vi "__SBR_Ana2.vi"(9 "SBRAクラスタ":T1={"データ配列"=array801x21[16821 elements], "Points"=801, "Th"=297.0, "Tc"=77.0, "LO(GHz)"=920.0, "Offset(mm)"=23.113, "Pos(mm)"=0.0, "P/V         V/P"=FALSE, "AUTOSAVE"=TRUE, "file_name"="", "パス"=path "", "header+(filename)"="A_"}) -> (0 "XYグラフ 6":cluster{"データ配列":dbl[], "データ配列":dbl[]}[](graph), 2 "XYグラフ 9":cluster{"データ配列":dbl[], "データ配列":dbl[]}[](graph), 3 "XYグラフ 5":cluster{"データ配列":dbl[], "データ配列":dbl[]}[](graph))   [LabVIEW 2017]
uses:
  <vilib>/Utility/file.llb/Read From Spreadsheet File (DBL).vi
  <vilib>/express/express arith-compare/Formula/XNode/ExpressFormulaBlockNode.xnode
panel:
  out "XYグラフ 8":cluster{"データ配列":dbl[], "データ配列":dbl[]}[](graph)
  in  "タブ制御器":T2(tab)
  out "XYグラフ":cluster{dbl[], dbl[]}[](graph)
  out "XYグラフ 4":cluster{"データ配列":dbl[], "データ配列":dbl[]}[](graph)
  out "XYグラフ 7":cluster{"データ配列":dbl[], "データ配列":dbl[]}[](graph)
  # "Port"
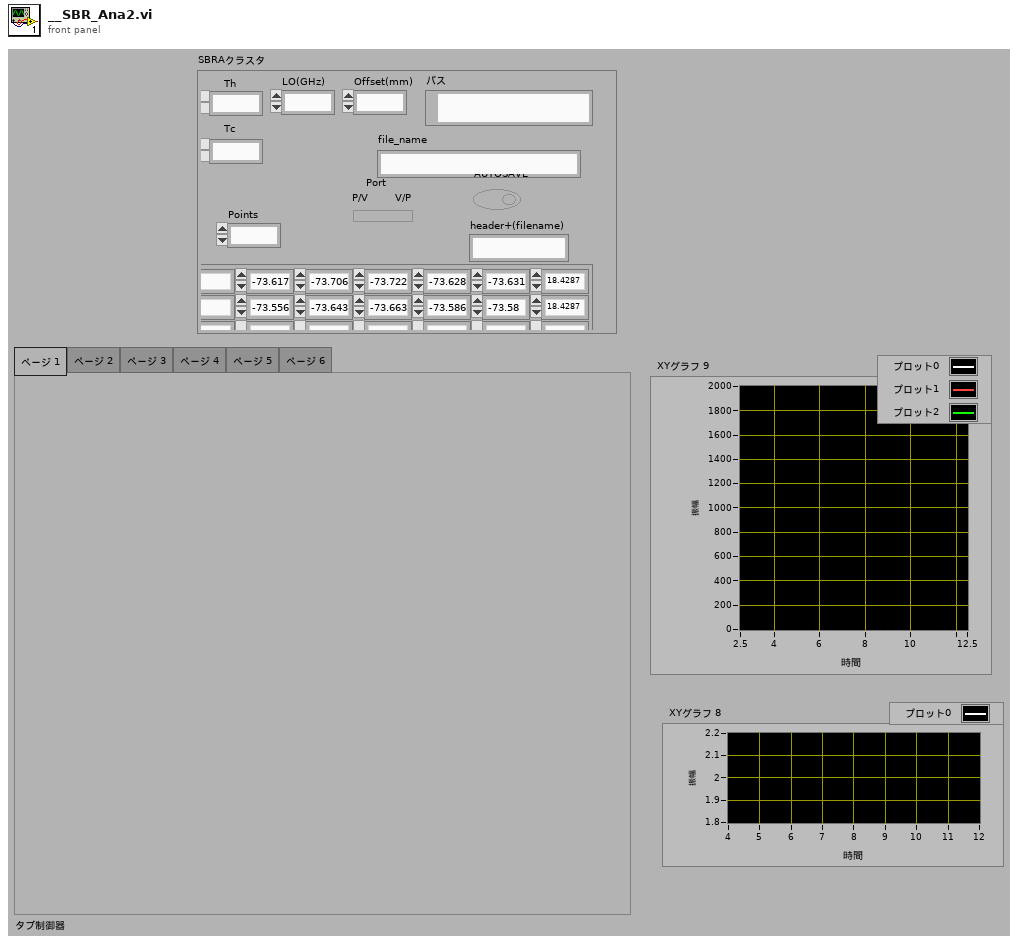
[diagram p1: front panel]
types:
  T1 = cluster{"データ配列":dbl[][], "Points":i32, "Th":dbl, "Tc":dbl, "LO(GHz)":dbl, "Offset(mm)":dbl, "Pos(mm)":dbl, "P/V         V/P":bool, "AUTOSAVE":bool, "file_name":string, "パス":path, "header+(filename)":string}
  T2 = enum32{"ページ 1", "ページ 2", "ページ 3", "ページ 4", "ページ 5", "ページ 6"}
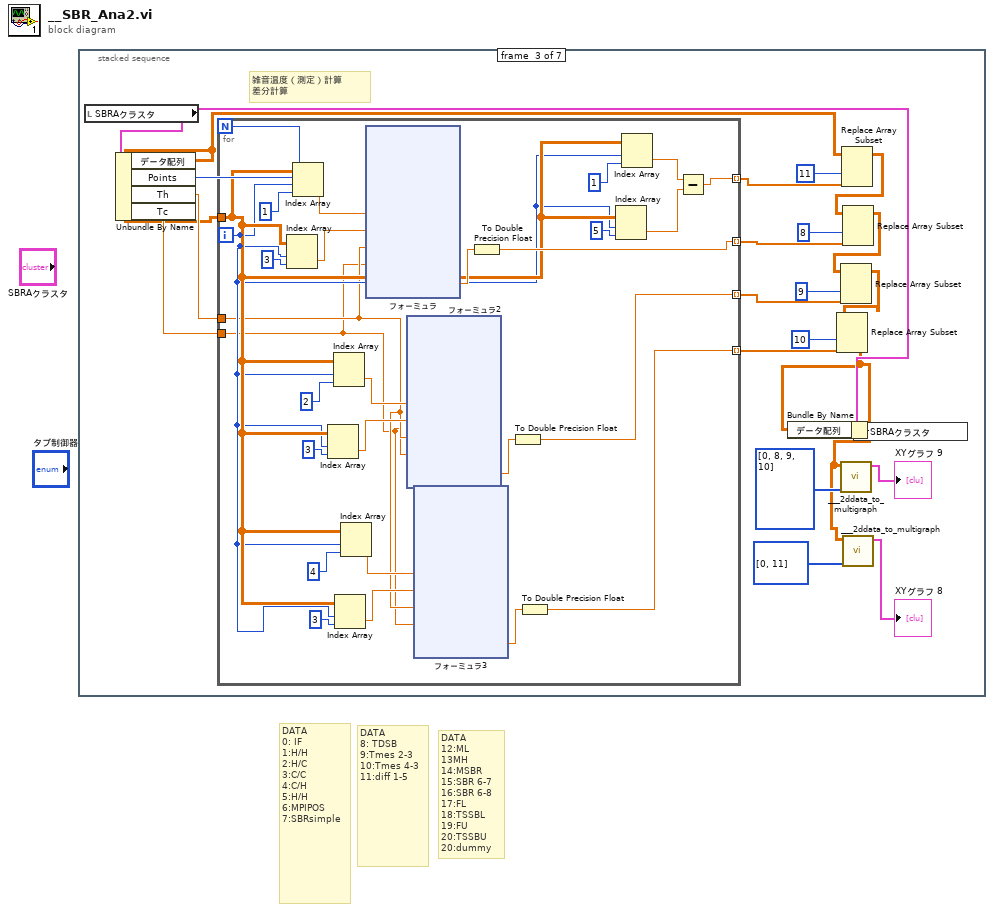
[diagram p0: block diagram]
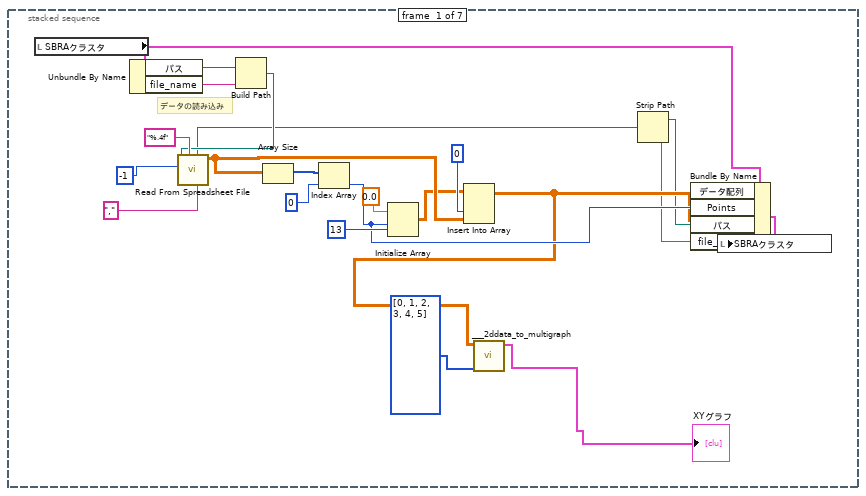
[diagram p2: hidden frame]
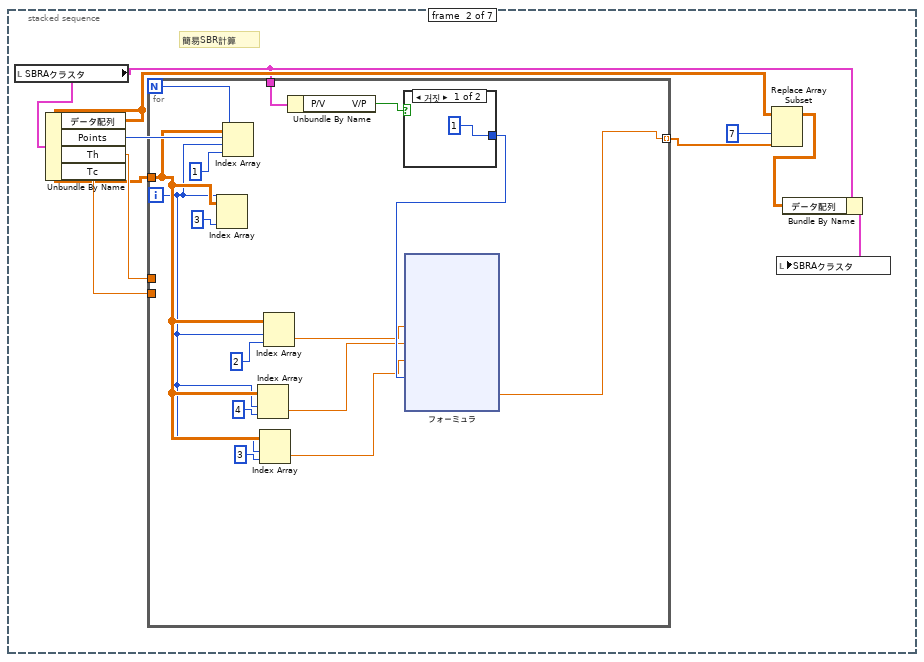
[diagram p3: hidden frame]
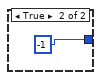
[diagram p4: hidden frame]
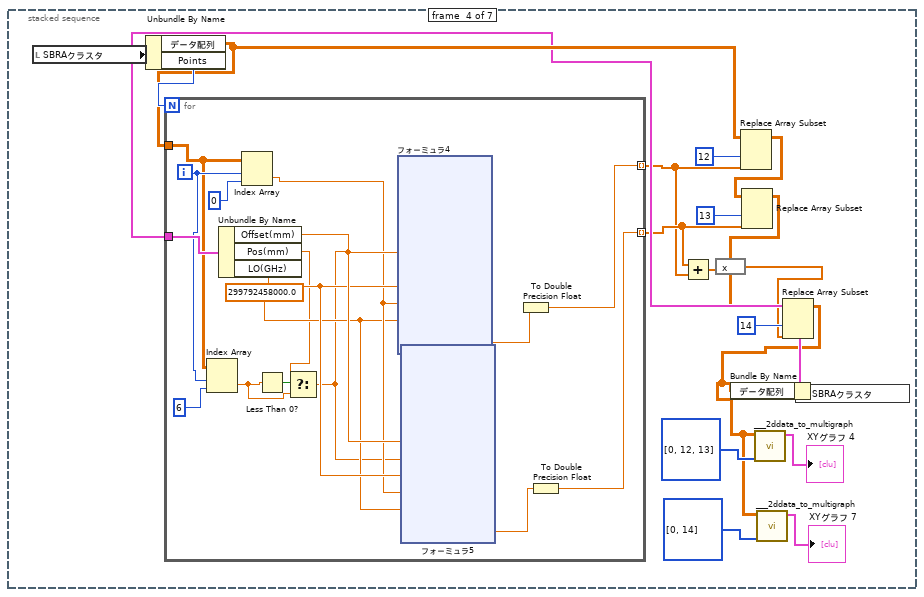
[diagram p5: hidden frame]
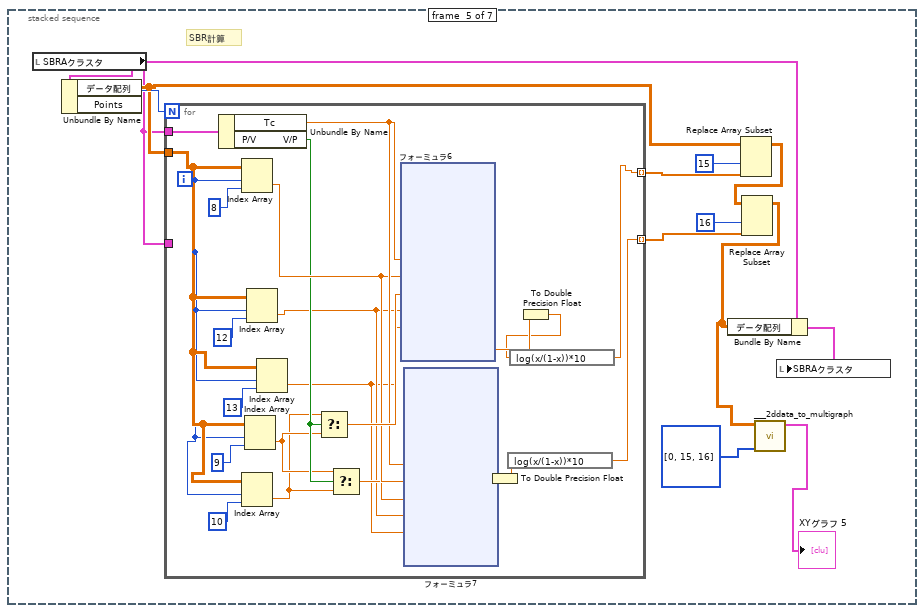
[diagram p6: hidden frame]
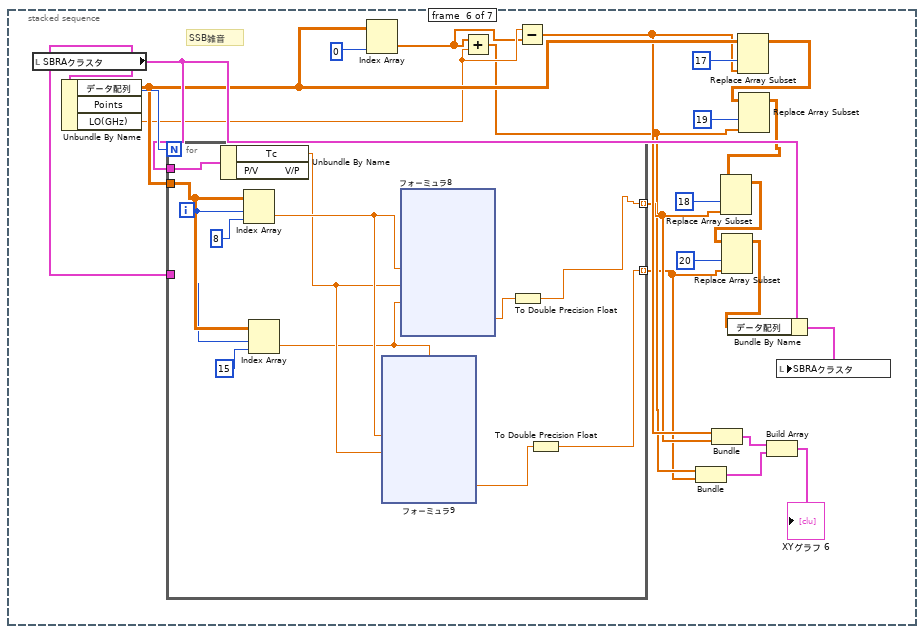
[diagram p7: hidden frame]
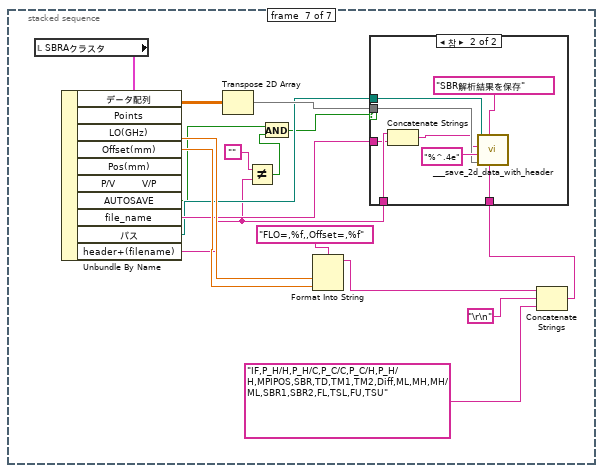
[diagram p8: hidden frame]
diagram:
  # "DATA\n12:ML\n13MH\n14:MSBR\n15:SBR 6-7\n16:SBR 6-8\n17:FL\n18:TSSBL\n19:FU\n20:TSSBU\n20:dummy"
  # "DATA\n8: TDSB\n9:Tmes 2-3\n10:Tmes 4-3\n11:diff 1-5"
  # "DATA\n0: IF\n1:H/H\n2:H/C\n3:C/C\n4:C/H\n5:H/H\n6:MPIPOS\n7:SBRsimple"
  n1 = stacked-sequence {
    frame #0 {
      # "データの読み込み"
      n2 = local read "SBRAクラスタ"() -> (w7:T1)
      n3 = Unbundle By Name(w7) -> ("パス"=w6:path, "file_name"=w5:string)
      n4 = Build Path(base path=w6, name or relative path=w5) -> (appended path=w4:path)
      n5 = call-poly <vilib>:"Read From Spreadsheet File.vi"("delimiter (\\t)"=",", "format (%.3f)"="%.4f", "number of rows (all:-1)"=-1, "file path (dialog if empty)"=w4) -> ("all rows"=w9:dbl[][], "new file path (Not A Path if cancelled)"=w1:path)  [unwired: 3 in, 3 out]
      n6 = Array Size(array=w9) -> (size(s)=w20:i32[])
      n7 = Index Array(array=w20, index=0) -> (element=w14:i32)
      n8 = Initialize Array(0.0, w14, 13) -> (w8:dbl[][])
      n9 = Insert Into Array(array=w8, index (col)=0, new element=w9) -> (w12:dbl[][])  [unwired: 1 in]
      n10 = call "___2ddata_to_multigraph.vi"("列"=i32[] [0, 1, 2, 3, 4, 5], "データ配列"=w12) -> ("XYグラフ"=→"XYグラフ":cluster{"データ配列":dbl[], "データ配列":dbl[]}[])  [unwired: 5 in]
      n11 = Strip Path(path=w1) -> (stripped path=w3:path, name=w2:string)
      n12 = Bundle By Name(cluster=w7, "データ配列"=w12, "Points"=w14, "パス"=w3, "file_name"=w2) -> (w15:T1)
      n13 = local write "SBRAクラスタ"(w15) -> ()
    }
    frame #1 {
      # "簡易SBR計算"
      n14 = local read "SBRAクラスタ"() -> (w24:T1)
      n15 = Unbundle By Name(w24) -> ("データ配列"=w28:dbl[][], "Points"=w31:i32, "Th"=w30:dbl, "Tc"=w29:dbl)
      n16 = for {
        N: w31 -> [_]
        tunnel: w28 -> [w40]
        tunnel: w30 -> [_]
        tunnel: w29 -> [_]
        tunnel: [w32] -> w25 mode=indexing
        tunnel: w24 -> [w38]
        i -> [w39]
        n17 = Index Array(array=w40, index (row)=w39, index (col)=3) -> ()  [unwired: 1 out]
        n18 = Index Array(array=w40, index (row)=w39, index (col)=1) -> ()  [unwired: 1 out]
        n19 = Index Array(array=w40, index (row)=w39, index (col)=4) -> (element=w34:dbl)
        n20 = Index Array(array=w40, index (row)=w39, index (col)=3) -> (element=w33:dbl)
        n21 = Index Array(array=w40, index (row)=w39, index (col)=2) -> (element=w35:dbl)
        n22 = Unbundle By Name(w38) -> ("P/V         V/P"=w37:bool)
        n23 = case shown="거짓" w37 {
          tunnel: [1 -1] -> w36
          frame False {
          }
          frame True {
          }
        }
        n24 = xnode "フォーミュラ"("PHC"=w35, "PCH"=w34, "PCC"=w33, "sig"=w36) -> ("結果"=w32:dbl)  [unwired: 1 in, 1 out]
      }
      n25 = Replace Array Subset(array=w28, new element=w25, index (col)=7) -> (w23:dbl[][])  [unwired: 1 in]
      n26 = Bundle By Name(cluster=w24, "データ配列"=w23) -> (w27:T1)
      n27 = local write "SBRAクラスタ"(w27) -> ()
    }
    frame #2 {
      # "雑音温度（測定）計算\n差分計算"
      n28 = local read "SBRAクラスタ"() -> (w79:T1)
      n29 = Unbundle By Name(w79) -> ("データ配列"=w80:dbl[][], "Points"=w83:i32, "Th"=w82:dbl, "Tc"=w81:dbl)
      n30 = for {
        N: w83 -> [_]
        tunnel: [w109] -> w73 mode=indexing
        tunnel: w80 -> [w92]
        tunnel: w82 -> [w85]
        tunnel: w81 -> [w84]
        tunnel: [w89] -> w76 mode=indexing
        tunnel: [w87] -> w68 mode=indexing
        tunnel: [w86] -> w67 mode=indexing
        i -> [w88]
        n31 = Index Array(array=w92, index (row)=w88, index (col)=3) -> (element=w106:dbl)
        n32 = Index Array(array=w92, index (row)=w88, index (col)=1) -> (element=w105:dbl)
        n33 = Index Array(array=w92, index (row)=w88, index (col)=3) -> (element=w101:dbl)
        n34 = Index Array(array=w92, index (row)=w88, index (col)=2) -> (element=w100:dbl)
        n35 = Index Array(array=w92, index (row)=w88, index (col)=3) -> (element=w96:dbl)
        n36 = Index Array(array=w92, index (row)=w88, index (col)=4) -> (element=w95:dbl)
        n37 = xnode "フォーミュラ"("ph"=w105, "pc"=w106, "th"=w85, "tc"=w84) -> ("結果"=w110:dbl)  [unwired: 1 in, 1 out]
        n38 = xnode "フォーミュラ2"("ph"=w100, "pc"=w101, "th"=w85, "tc"=w84) -> ("結果"=w104:dbl)  [unwired: 1 in, 1 out]
        n39 = xnode "フォーミュラ3"("ph"=w95, "pc"=w96, "th"=w85, "tc"=w84) -> ("結果"=w99:dbl)  [unwired: 1 in, 1 out]
        n40 = To Double Precision Float(number=w110) -> (double precision float=w109:dbl)
        n41 = To Double Precision Float(number=w104) -> (double precision float=w87:dbl)
        n42 = To Double Precision Float(number=w99) -> (double precision float=w86:dbl)
        n43 = Index Array(array=w92, index (row)=w88, index (col)=5) -> (element=w90:dbl)
        n44 = Index Array(array=w92, index (row)=w88, index (col)=1) -> (element=w91:dbl)
        n45 = Subtract(x=w91, y=w90) -> (x-y=w89:dbl)
      }
      n46 = Replace Array Subset(array=w80, new element=w76, index (col)=11) -> (w74:dbl[][])  [unwired: 1 in]
      n47 = Replace Array Subset(array=w74, new element=w73, index (col)=8) -> (w71:dbl[][])  [unwired: 1 in]
      n48 = Replace Array Subset(array=w71, new element=w68, index (col)=9) -> (w69:dbl[][])  [unwired: 1 in]
      n49 = Replace Array Subset(array=w69, new element=w67, index (col)=10) -> (w63:dbl[][])  [unwired: 1 in]
      n50 = Bundle By Name(cluster=w79, "データ配列"=w63) -> (w78:T1)
      n51 = call "___2ddata_to_multigraph.vi"("列"=i32[] [0, 8, 9, 10], "データ配列"=w63) -> ("XYグラフ"=→"XYグラフ 9":cluster{"データ配列":dbl[], "データ配列":dbl[]}[])  [unwired: 5 in]
      n52 = call "___2ddata_to_multigraph.vi"("列"=i32[] [0, 11], "データ配列"=w63) -> ("XYグラフ"=→"XYグラフ 8":cluster{"データ配列":dbl[], "データ配列":dbl[]}[])  [unwired: 5 in]
      n53 = local write "SBRAクラスタ"(w78) -> ()
    }
    frame #3 {
      n54 = local read "SBRAクラスタ"() -> (w165:T1)
      n55 = Unbundle By Name(w165) -> ("データ配列"=w166:dbl[][], "Points"=w170:i32)
      n56 = for {
        N: w170 -> [_]
        tunnel: w166 -> [w175]
        tunnel: w165 -> [w186]
        tunnel: [w179] -> w160 mode=indexing
        tunnel: [w178] -> w161 mode=indexing
        i -> [w176]
        w182 = 299792458000.0
        n57 = Index Array(array=w175, index (row)=w176, index (col)=6) -> (element=w172:dbl)
        n58 = Unbundle By Name(w186) -> ("Offset(mm)"=w185:dbl, "Pos(mm)"=w173:dbl, "LO(GHz)"=w184:dbl)
        n59 = Index Array(array=w175, index (row)=w176, index (col)=0) -> (element=w183:dbl)
        n60 = Less Than 0?(x=w172) -> (x < 0?=w174:bool)
        n61 = Select(t=w173, s=w174, f=w172) -> (s? t:f=w171:dbl)
        n62 = xnode "フォーミュラ4"("OS"=w185, "POS"=w171, "LO"=w184, "IF"=w183, "VC"=w182) -> ("結果"=w181:dbl)  [unwired: 1 in, 1 out]
        n63 = xnode "フォーミュラ5"("OS"=w185, "POS"=w171, "LO"=w184, "IF"=w183, "VC"=w182) -> ("結果"=w180:dbl)  [unwired: 1 in, 1 out]
        n64 = To Double Precision Float(number=w181) -> (double precision float=w179:dbl)
        n65 = To Double Precision Float(number=w180) -> (double precision float=w178:dbl)
      }
      n66 = Add(x=w161, y=w160) -> (x+y=w159:dbl[])
      n67 = expression code="x"(w159) -> (w157:dbl[])
      n68 = Replace Array Subset(array=w166, new element=w160, index (col)=12) -> (w167:dbl[][])  [unwired: 1 in]
      n69 = Replace Array Subset(array=w167, new element=w161, index (col)=13) -> (w156:dbl[][])  [unwired: 1 in]
      n70 = Replace Array Subset(array=w156, new element=w157, index (col)=14) -> (w153:dbl[][])  [unwired: 1 in]
      n71 = Bundle By Name(cluster=w165, "データ配列"=w153) -> (w164:T1)
      n72 = call "___2ddata_to_multigraph.vi"("列"=i32[] [0, 12, 13], "データ配列"=w153) -> ("XYグラフ"=→"XYグラフ 4":cluster{"データ配列":dbl[], "データ配列":dbl[]}[])  [unwired: 5 in]
      n73 = call "___2ddata_to_multigraph.vi"("列"=i32[] [0, 14], "データ配列"=w153) -> ("XYグラフ"=→"XYグラフ 7":cluster{"データ配列":dbl[], "データ配列":dbl[]}[])  [unwired: 5 in]
      n74 = local write "SBRAクラスタ"(w164) -> ()
    }
    frame #4 {
      # "SBR計算"
      n75 = local read "SBRAクラスタ"() -> (w221:T1)
      n76 = Unbundle By Name(w221) -> ("データ配列"=w227:dbl[][], "Points"=w231:i32)
      n77 = for {
        N: w231 -> [_]
        tunnel: w227 -> [w247]
        tunnel: w221 -> [_]
        tunnel: [w237] -> w226 mode=indexing
        tunnel: [w236] -> w225 mode=indexing
        tunnel: w221 -> [w249]
        i -> [w246]
        n78 = Unbundle By Name(w249) -> ("Tc"=w243:dbl, "P/V         V/P"=w241:bool)
        n79 = Index Array(array=w247, index (row)=w246, index (col)=8) -> (element=w242:dbl)
        n80 = Index Array(array=w247, index (row)=w246, index (col)=10) -> (element=w232:dbl)
        n81 = Index Array(array=w247, index (row)=w246, index (col)=9) -> (element=w233:dbl)
        n82 = Index Array(array=w247, index (row)=w246, index (col)=12) -> (element=w235:dbl)
        n83 = Index Array(array=w247, index (row)=w246, index (col)=13) -> (element=w234:dbl)
        n84 = Select(t=w232, s=w241, f=w233) -> (s? t:f=w245:dbl)
        n85 = Select(t=w233, s=w241, f=w232) -> (s? t:f=w240:dbl)
        n86 = xnode "フォーミュラ6"("TC"=w243, "TD"=w242, "TM"=w245, "ML"=w235, "MU"=w234) -> ("結果"=w253:dbl)  [unwired: 1 in, 1 out]
        n87 = xnode "フォーミュラ7"("TC"=w243, "TD"=w242, "TM"=w240, "ML"=w235, "MU"=w234) -> ("結果"=w239:dbl)  [unwired: 1 in, 1 out]
        n88 = To Double Precision Float(number=w239) -> (double precision float=w238:dbl)
        n89 = expression code="log(x/(1-x))*10"(w238) -> (w236:dbl)
        n90 = To Double Precision Float(number=w253) -> (double precision float=w244:dbl)
        n91 = expression code="log(x/(1-x))*10"(w244) -> (w237:dbl)
      }
      n92 = Replace Array Subset(array=w227, new element=w226, index (col)=15) -> (w228:dbl[][])  [unwired: 1 in]
      n93 = Replace Array Subset(array=w228, new element=w225, index (col)=16) -> (w222:dbl[][])  [unwired: 1 in]
      n94 = Bundle By Name(cluster=w221, "データ配列"=w222) -> (w224:T1)
      n95 = call "___2ddata_to_multigraph.vi"("列"=i32[] [0, 15, 16], "データ配列"=w222) -> ("XYグラフ"=→"XYグラフ 5":cluster{"データ配列":dbl[], "データ配列":dbl[]}[])  [unwired: 5 in]
      n96 = local write "SBRAクラスタ"(w224) -> ()
    }
    frame #5 {
      # "SSB雑音"
      n97 = local read "SBRAクラスタ"() -> (w303:T1)
      n98 = Unbundle By Name(w303) -> ("データ配列"=w301:dbl[][], "Points"=w308:i32, "LO(GHz)"=w300:dbl)
      n99 = for {
        N: w308 -> [_]
        tunnel: w301 -> [w317]
        tunnel: w303 -> [_]
        tunnel: [w309] -> w292 mode=indexing
        tunnel: [w310] -> w290 mode=indexing
        tunnel: w303 -> [w318]
        i -> [w316]
        n100 = Unbundle By Name(w318) -> ("Tc"=w313:dbl)  [unwired: 1 out]
        n101 = Index Array(array=w317, index (row)=w316, index (col)=8) -> (element=w314:dbl)
        n102 = Index Array(array=w317, index (row)=w316, index (col)=15) -> (element=w312:dbl)
        n103 = xnode "フォーミュラ9"("TD"=w314, "TC"=w313, "SBR"=w312) -> ("結果"=w311:dbl)  [unwired: 1 in, 1 out]
        n104 = xnode "フォーミュラ8"("TD"=w314, "TC"=w313, "SBR"=w312) -> ("結果"=w315:dbl)  [unwired: 1 in, 1 out]
        n105 = To Double Precision Float(number=w315) -> (double precision float=w309:dbl)
        n106 = To Double Precision Float(number=w311) -> (double precision float=w310:dbl)
      }
      n107 = Index Array(array=w301, index (col)=0) -> (element=w299:dbl[])  [unwired: 1 in]
      n108 = Add(x=w299, y=w300) -> (x+y=w291:dbl[])
      n109 = Subtract(x=w300, y=w299) -> (x-y=w293:dbl[])
      n110 = Bundle(w291, w290) -> (w288:cluster{dbl[], dbl[]})  [unwired: 1 in]
      n111 = Bundle(w293, w292) -> (w289:cluster{dbl[], dbl[]})  [unwired: 1 in]
      n112 = Replace Array Subset(array=w301, new element=w293, index (col)=17) -> (w305:dbl[][])  [unwired: 1 in]
      n113 = Replace Array Subset(array=w305, new element=w291, index (col)=19) -> (w296:dbl[][])  [unwired: 1 in]
      n114 = Replace Array Subset(array=w296, new element=w292, index (col)=18) -> (w295:dbl[][])  [unwired: 1 in]
      n115 = Replace Array Subset(array=w295, new element=w290, index (col)=20) -> (w294:dbl[][])  [unwired: 1 in]
      n116 = Bundle By Name(cluster=w303, "データ配列"=w294) -> (w304:T1)
      n117 = Build Array(w289, w288) -> (→"XYグラフ 6":cluster{dbl[], dbl[]}[])
      n118 = local write "SBRAクラスタ"(w304) -> ()
    }
    frame #6 {
      n119 = local read "SBRAクラスタ"() -> (w361:T1)
      n120 = Unbundle By Name(w361) -> ("データ配列"=w360:dbl[][], "LO(GHz)"=w359:dbl, "Offset(mm)"=w358:dbl, "AUTOSAVE"=w346:bool, "file_name"=w351:string, "パス"=w350:path, "header+(filename)"=w349:string)  [unwired: 3 out]
      n121 = Transpose 2D Array(2D array=w360) -> (transposed array=w354:dbl[][])
      n122 = Not Equal?(x="", y=w349) -> (x != y?=w347:bool)
      n123 = And(x=w346, y=w347) -> (x .and. y?=w345:bool)
      n124 = Format Into String(format string="FLO=,%f,,Offset=,%f", w359, w358) -> (resulting string=w352:string)  [unwired: 2 in, 1 out]
      n125 = Concatenate Strings(w352, "\r\n", "IF,P_H/H,P_H/C,P_C/C,P_C/H,P_H/H,MPIPOS,SBR,TD,TM1,TM2,Diff,ML,MH,MH/ML,SBR1,SBR2,FL,TSL,FU,TSU") -> (w355:string)
      n126 = case shown="참" w345 {
        tunnel: w355 -> [_ w368]
        tunnel: w354 -> [_ w367]
        tunnel: w349 -> [_ w365]
        tunnel: w351 -> [_ w364]
        tunnel: w350 -> [_ w362]
        frame False {
        }
        frame True {
          n127 = Concatenate Strings(w365, w364) -> (w363:string)
          n128 = call "___save_2d_data_with_header.vi"("ヘッダー"=w368, "プロンプト"="SBR解析結果を保存", "配列"=w367, "形式"="%^.4e", "file_name"=w363, "パス"=w362) -> ()  [unwired: 5 in, 1 out]
        }
      }
    }
  }
